vi "Set Scaling Parameters (Table).vi"(0 "session in":refnum<k21>, 1 "serial number":string, 2 "password":string, 5 "physical channel":refnum<k21>="$DefaultPhysChans", 7 "scaled values":dbl[](array[numeric]), 9 "pre-scaled values":dbl[](array[numeric]), 11 "error in (no error)":errorcluster, 12 "coercion":i32(ring) items=["Interpolate", "RoundToNearest", "Strict"]) -> (4 "session out":refnum<k21>, 6 "physical channel out":refnum<k21>, 15 "error out":errorcluster)   [LabVIEW 2020, in "SLSC.lvlib"]
doc: "Sets scaling parameters for a table scale that maps an array of pre-scaled values to an array of corresponding scaled values."
uses:
  <vilib>/SLSC/SLSC.lvlib
  nislsclvapi.dll
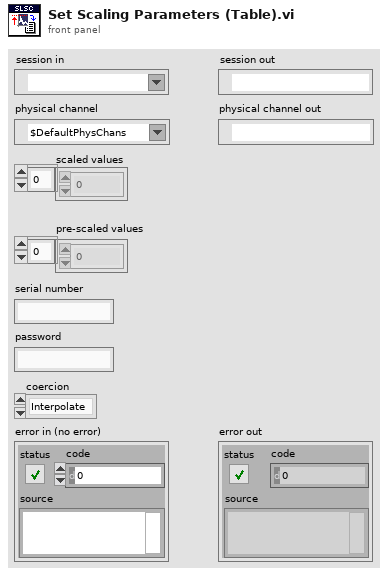
[diagram p1: front panel]
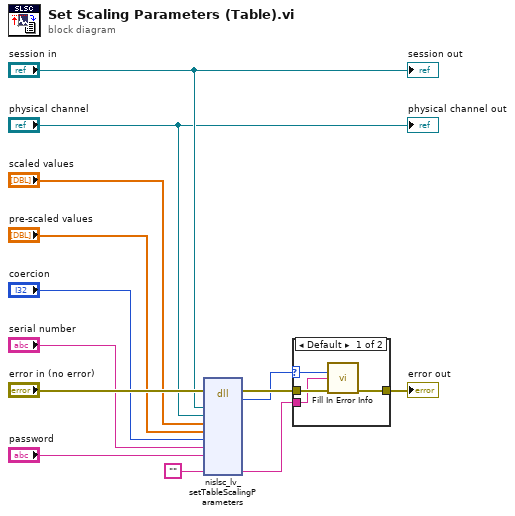
[diagram p0: block diagram]
diagram:
  n1 = dll-call lib="nislsclvapi.*" fn="nislsc_lv_setTableScalingParameters"(error in="error in (no error)", "session"="session in", "physical channel"="physical channel", "scaledValues"="scaled values", "prescaleValues"="pre-scaled values", "coercion"="coercion", "serialNum"="serial number", "password"="password", "extendedErrorInfo"="") -> (error out=w4:errorcluster, "return type"=w2:i32, "extendedErrorInfo"=w3:string)  [unwired: 11 in, 1 out]
  n2 = case shown="Default" w2 {
    selector: w2 -> [w14 _]
    tunnel: w3 -> [w15 _]
    tunnel: w4 -> [w17 w18]
    tunnel: [w16 w18] -> w1
    frame Default {
      n3 = call <vilib>:"Fill In Error Info.vi"("status code"=w14, "extended error info"=w15, "error in"=w17) -> ("error out"=w16:errorcluster)  [unwired: 12 in]
    }
    frame 0 {
    }
  }
  "error out" <- w1
  "session out" <- "session in"
  "physical channel out" <- "physical channel"
